vi "MTS_ReadMSW.vi"(8 "error in (no error)":errorcluster, 11 "Workspace Path":path) -> (0 "error out":errorcluster, 1 "Created":string, 2 "Comment":string, 3 "Files in Workspace":T1(array[cluster]))   [LabVIEW 2013]
uses:
  <vilib>/Utility/config.llb/Read Key (String).vi
  <vilib>/Utility/config.llb/Read Key (Path).vi
  <vilib>/Utility/config.llb/Read Key (I32).vi
  <vilib>/Utility/config.llb/Read Key (Double).vi
  <vilib>/Utility/config.llb/Read Key (U32).vi
  <vilib>/Utility/config.llb/NI_LVConfig.lvlib
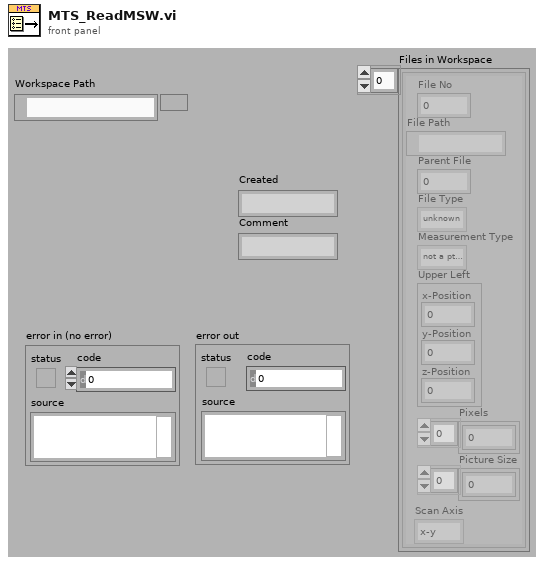
[diagram p1: front panel]
types:
  T1 = cluster{"File No":i32, "File Path":path, "Parent File":i32, "File Type":enum16{"unknown", "pt3 File", "png Image", "bmp Image"}, "Measurement Type":enum16{"not a pt3 File", "Image File", "Point Measurement", "Auto Point", "Line Scan", "Grid Scan"}, "Upper Left":cluster{"x-Position":dbl, "y-Position":dbl, "z-Position":dbl}, "Pixels":i32[], "Picture Size":dbl[], "Scan Axis":enum32{"x-y", "x-z", "y-z"}}[]
  T2 = cluster{"File No":i32, "File Path":path, "Parent File":i32, "File Type":enum16{"unknown", "pt3 File", "png Image", "bmp Image"}, "Measurement Type":enum16{"not a pt3 File", "Image File", "Point Measurement", "Auto Point", "Line Scan", "Grid Scan"}, "Upper Left":cluster{"x-Position":dbl, "y-Position":dbl, "z-Position":dbl}, "Pixels":u16[], "Picture Size":dbl[], "Scan Axis":enum32{"x-y", "x-z", "y-z"}}
  T3 = typedef "NI_LVConfig.lvlib/Config Data RefNum.ctl" = refnum<k1>
  T4 = cluster{"File No":i32, "File Path":path, "Parent File":i32, "File Type":enum16{"unknown", "pt3 File", "png Image", "bmp Image"}, "Measurement Type":enum16{"not a pt3 File", "Image File", "Point Measurement", "Auto Point", "Line Scan", "Grid Scan"}, "Upper Left":cluster{"x-Position":dbl, "y-Position":dbl, "z-Position":dbl}, "Pixels":u16[], "Picture Size":dbl[], "Scan Axis":enum32{"x-y", "x-z", "y-z"}}[]
  T5 = enum16{"not a pt3 File", "Image File", "Point Measurement", "Auto Point", "Line Scan", "Grid Scan"}
  T6 = enum16{"unknown", "pt3 File", "png Image", "bmp Image"}
  T7 = cluster{i32, "value":path, "value":i32, "File Type":enum16{"unknown", "pt3 File", "png Image", "bmp Image"}, "Measurement Type":enum16{"not a pt3 File", "Image File", "Point Measurement", "Auto Point", "Line Scan", "Grid Scan"}, cluster{"value":dbl, "value":dbl, "value":dbl}, i32[], dbl[], "value":u32}
  T8 = cluster{"File No":i32, "value":path, "value":i32, "File Type":enum16{"unknown", "pt3 File", "png Image", "bmp Image"}, "Measurement Type":enum16{"not a pt3 File", "Image File", "Point Measurement", "Auto Point", "Line Scan", "Grid Scan"}, "Upper Left":cluster{"value":dbl, "value":dbl, "value":dbl}, "Pixels":i32[], "Picture Size":dbl[], "value":u32}[]
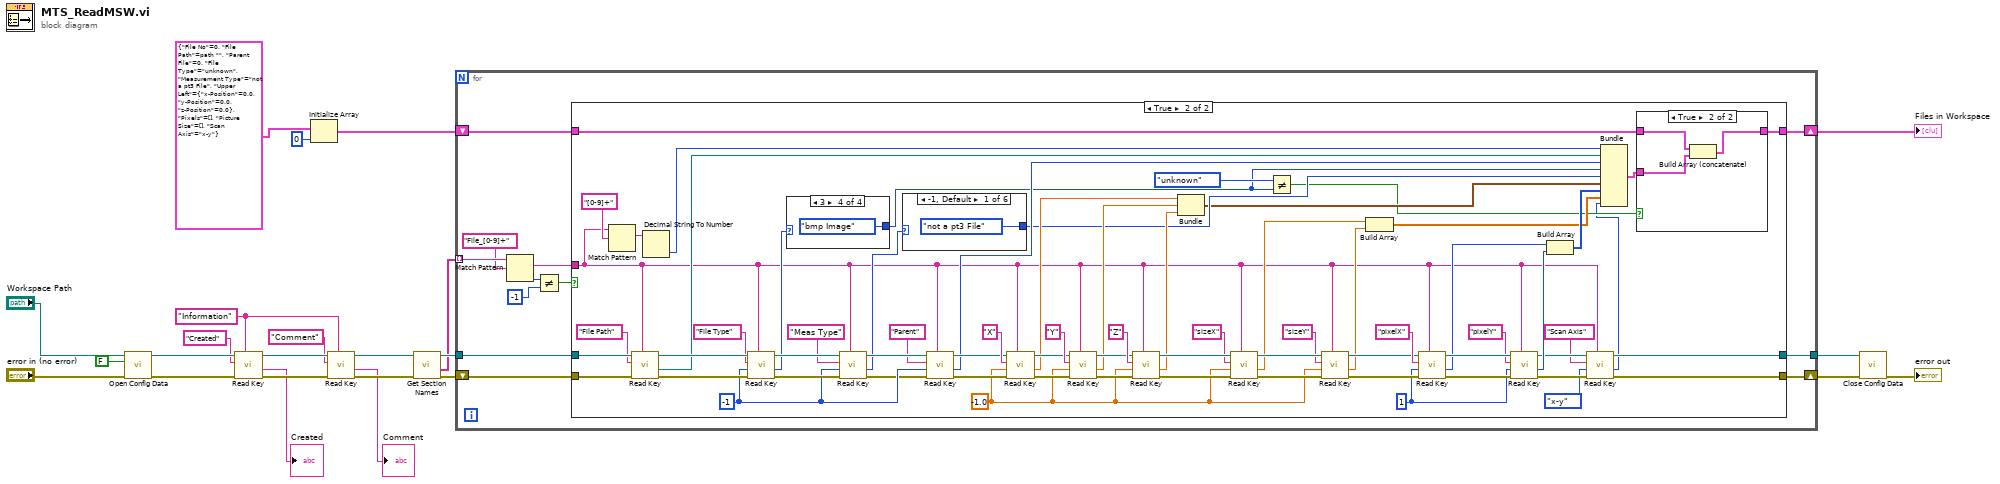
[diagram p0: block diagram]
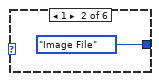
[diagram p4: hidden frame]
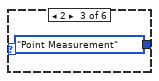
[diagram p5: hidden frame]
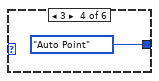
[diagram p6: hidden frame]
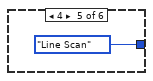
[diagram p7: hidden frame]
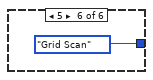
[diagram p8: hidden frame]
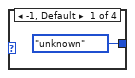
[diagram p9: hidden frame]
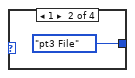
[diagram p10: hidden frame]
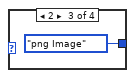
[diagram p11: hidden frame]
diagram:
  w16 = "Information" ("section")
  n1 = call <vilib>:"Open Config Data.vi"("error in (no error)"="error in (no error)", "create file if necessary (T)"=FALSE, "configuration file path"="Workspace Path") -> ("error out"=w21:errorcluster, "refnum"=w20:T3)  [unwired: 6 in, 1 out]
  n2 = call-poly <vilib>:"Read Key.vi"("section"=w16, "error in (no error)"=w21, "key"="Created", "refnum"=w20) -> ("error out"=w18:errorcluster, "value"=→"Created":string, "refnum out"=w17:T3)  [unwired: 4 in, 1 out]
  n3 = Initialize Array(T2 {"File No"=0, "File Path"=path "", "Parent File"=0, "File Type"=enum."unknown", "Measurement Type"=enum."not a pt3 File", "Upper Left"={"x-Position"=0.0, "y-Position"=0.0, "z-Position"=0.0}, "Pixels"=[], "Picture Size"=[], "Scan Axis"=enum."x-y"} ("Cluster"), 0 ("dimension size")) -> (w4:T4)
  n4 = call-poly <vilib>:"Read Key.vi"("section"=w16, "error in (no error)"=w18, "key"="Comment", "refnum"=w17) -> ("error out"=w14:errorcluster, "value"=→"Comment":string, "refnum out"=w13:T3)  [unwired: 4 in, 1 out]
  n5 = call <vilib>:"Get Section Names.vi"("error in (no error)"=w14, "refnum"=w13) -> ("error out"=w12:errorcluster, "section names"=w10:string[], "refnum out"=w11:T3)  [unwired: 7 in]
  n6 = for {
    shift-right: [w28] -> w9
    shift-left: w12 -> [w30]
    tunnel: w11 -> [w29]
    tunnel: w10 -> [w36] mode=indexing
    tunnel: [w27] -> w8
    shift-right: [w25] -> w1
    shift-left: w4 -> [w26]
    n7 = Match Pattern(string=w36, regular expression="File_[0-9]+") -> (match substring=w31:string, offset past match=w34:i32)  [unwired: 1 in, 2 out]
    n8 = Not Equal?(x=w34, y=-1) -> (x != y?=w32:bool)
    n9 = case shown="True" w32 {
      tunnel: w31 -> [_ w41]
      tunnel: w30 -> [w39 w107]
      tunnel: w29 -> [w38 w106]
      tunnel: [w39 w46] -> w28
      tunnel: [w38 w44] -> w27
      tunnel: w26 -> [w37 w50]
      tunnel: [w37 w48] -> w25
      frame False {
      }
      frame True {
        w70 = 1 ("default value")
        w71 = -1.0 ("default value")
        w97 = -1 ("default value")
        n10 = Match Pattern(string=w41, regular expression="[0-9]+") -> (match substring=w98:string)  [unwired: 1 in, 3 out]
        n11 = call-poly <vilib>:"Read Key.vi"("section"=w41, "error in (no error)"=w107, "key"="File Path", "refnum"=w106) -> ("error out"=w104:errorcluster, "value"=w58:path, "refnum out"=w103:T3)  [unwired: 4 in, 1 out]
        n12 = Decimal String To Number(string=w98) -> (number=w59:i32)  [unwired: 2 in, 1 out]
        n13 = call-poly <vilib>:"Read Key.vi"("section"=w41, "error in (no error)"=w104, "default value"=w97, "key"="File Type", "refnum"=w103) -> ("error out"=w101:errorcluster, "value"=w62:i32, "refnum out"=w100:T3)  [unwired: 3 in, 1 out]
        n14 = case shown="3" w62 {
          tunnel: [T6."unknown" ("File Type") T6."pt3 File" ("File Type") T6."png Image" ("File Type") T6."bmp Image" ("File Type")] -> w56
          frame -1, Default {
          }
          frame 1 {
          }
          frame 2 {
          }
          frame 3 {
          }
        }
        n15 = call-poly <vilib>:"Read Key.vi"("section"=w41, "error in (no error)"=w101, "default value"=w97, "key"="Meas Type", "refnum"=w100) -> ("error out"=w96:errorcluster, "value"=w61:i32, "refnum out"=w95:T3)  [unwired: 3 in, 1 out]
        n16 = case shown="-1, Default" w61 {
          tunnel: [T5."not a pt3 File" ("Measurement Type") T5."Image File" ("Measurement Type") T5."Point Measurement" ("Measurement Type") T5."Auto Point" ("Measurement Type") T5."Line Scan" ("Measurement Type") T5."Grid Scan" ("Measurement Type")] -> w55
          frame -1, Default {
          }
          frame 1 {
          }
          frame 2 {
          }
          frame 3 {
          }
          frame 4 {
          }
          frame 5 {
          }
        }
        n17 = call-poly <vilib>:"Read Key.vi"("section"=w41, "error in (no error)"=w96, "default value"=w97, "key"="Parent", "refnum"=w95) -> ("error out"=w92:errorcluster, "value"=w57:i32, "refnum out"=w86:T3)  [unwired: 3 in, 1 out]
        n18 = call-poly <vilib>:"Read Key.vi"("section"=w41, "error in (no error)"=w92, "default value"=w71, "key"="X", "refnum"=w86) -> ("error out"=w91:errorcluster, "value"=w65:dbl, "refnum out"=w85:T3)  [unwired: 3 in, 1 out]
        n19 = call-poly <vilib>:"Read Key.vi"("section"=w41, "error in (no error)"=w91, "default value"=w71, "key"="Y", "refnum"=w85) -> ("error out"=w90:errorcluster, "value"=w64:dbl, "refnum out"=w84:T3)  [unwired: 3 in, 1 out]
        n20 = call-poly <vilib>:"Read Key.vi"("section"=w41, "error in (no error)"=w90, "default value"=w71, "key"="Z", "refnum"=w84) -> ("error out"=w83:errorcluster, "value"=w63:dbl, "refnum out"=w81:T3)  [unwired: 3 in, 1 out]
        n21 = Bundle("value"=w65, "value"=w64, "value"=w63) -> (w54:cluster{"value":dbl, "value":dbl, "value":dbl})  [unwired: 1 in]
        n22 = call-poly <vilib>:"Read Key.vi"("section"=w41, "error in (no error)"=w83, "default value"=w71, "key"="sizeX", "refnum"=w81) -> ("error out"=w82:errorcluster, "value"=w69:dbl, "refnum out"=w80:T3)  [unwired: 3 in, 1 out]
        n23 = Not Equal?(x=enum16{"unknown", "pt3 File", "png Image"}."unknown" ("File Type"), y=w56) -> (x != y?=w51:bool)
        n24 = call-poly <vilib>:"Read Key.vi"("section"=w41, "error in (no error)"=w82, "default value"=w71, "key"="sizeY", "refnum"=w80) -> ("error out"=w73:errorcluster, "value"=w68:dbl, "refnum out"=w72:T3)  [unwired: 3 in, 1 out]
        n25 = Build Array(w69, w68) -> (w52:dbl[])
        n26 = call-poly <vilib>:"Read Key.vi"("section"=w41, "error in (no error)"=w73, "default value"=w70, "key"="pixelX", "refnum"=w72) -> ("error out"=w77:errorcluster, "value"=w67:i32, "refnum out"=w76:T3)  [unwired: 3 in, 1 out]
        n27 = call-poly <vilib>:"Read Key.vi"("section"=w41, "error in (no error)"=w77, "default value"=w70, "key"="pixelY", "refnum"=w76) -> ("error out"=w47:errorcluster, "value"=w66:i32, "refnum out"=w45:T3)  [unwired: 3 in, 1 out]
        n28 = Build Array(w67, w66) -> (w53:i32[])
        n29 = call-poly <vilib>:"Read Key.vi"("section"=w41, "error in (no error)"=w47, "default value"=enum32{"x-y", "x-z", "y-z"}."x-y" ("Scan Axis"), "key"="Scan Axis", "refnum"=w45) -> ("error out"=w46:errorcluster, "value"=w40:u32, "refnum out"=w44:T3)  [unwired: 3 in, 1 out]
        n30 = Bundle(w59, "value"=w58, "value"=w57, "File Type"=w56, "Measurement Type"=w55, w54, w53, w52, "value"=w40) -> (w49:T7)  [unwired: 1 in]
        n31 = case shown="True" w51 {
          tunnel: w50 -> [w108 w111]
          tunnel: w49 -> [_ w110]
          tunnel: [w108 w109] -> w48
          frame False {
          }
          frame True {
            n32 = Build Array (concatenate)(w111, w110) -> (w109:T8)
          }
        }
      }
    }
  }
  "Files in Workspace" <- w1
  n33 = call <vilib>:"Close Config Data.vi"("error in (no error)"=w9, "refnum"=w8) -> ("error out"=→"error out":errorcluster)  [unwired: 8 in, 1 out]
